vi "FTW-Message-Destroy.vi"(0 "FTW Lossy Message":refnum<class "FTW-Message-Lossy.lvclass">, 11 "error in":errorcluster) -> (15 "error out":errorcluster)   [LabVIEW 2013, in "FTW-Message-Lossy.lvclass"]
uses:
  FTW-Message-Lossy.lvclass
  FTW-Message-Lossy.lvclass/FTW-Message-Lossy.ctl
panel:
  # "Inputs"
  # "Outputs"
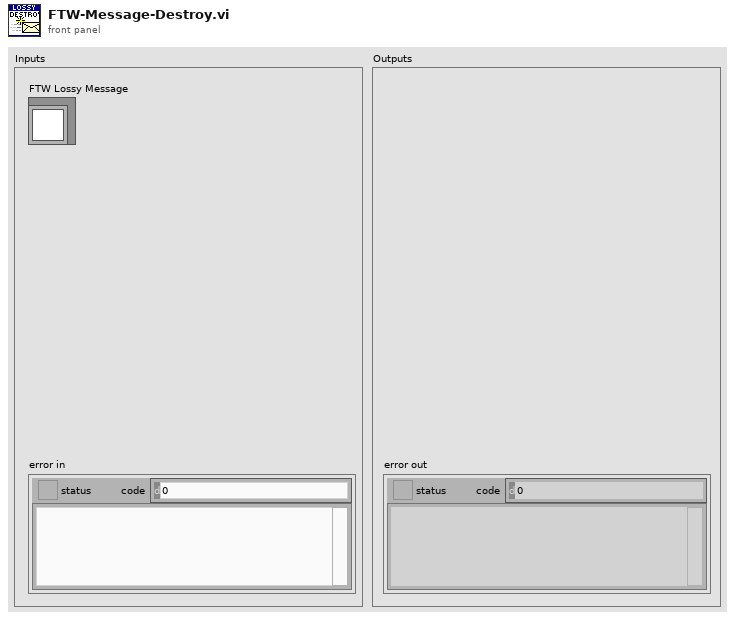
[diagram p1: front panel]
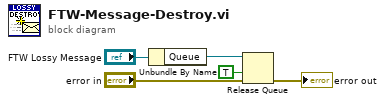
[diagram p0: block diagram]
diagram:
  n1 = Unbundle By Name("FTW Lossy Message") -> ("Queue"=w2:refnum<queue>)
  n2 = Release Queue(queue=w2, force destroy? (F)=TRUE, error in (no error)="error in") -> (error out=→"error out":errorcluster)  [unwired: 2 out]
